vi "Power_spectrum.vi"(0 "U":dbl[](array[numeric]) format="%.2f", 2 "Sampling frequency":dbl format="%.2f", 3 "Spectrum input array":dbl[](array[numeric]) format="%.2f", 4 "Block No":i32=1) -> (5 "dF":dbl, 6 "SingleBlockSpectrum":dbl[](array[numeric]) format="%.2f", 7 "Spectrum Accumulator array":dbl[](array[numeric]) format="%.2f")   [LabVIEW 2015]
uses:
  <vilib>/Analysis/2dsp.llb/Power Spectrum (DBL).vi
  <vilib>/Analysis/baseanly.llb/Mean.vi
  <vilib>/Analysis/baseanly.llb/Mean (DBL).vi
  <vilib>/Analysis/NI_AALPro.lvlib
panel:
  out "size":i32
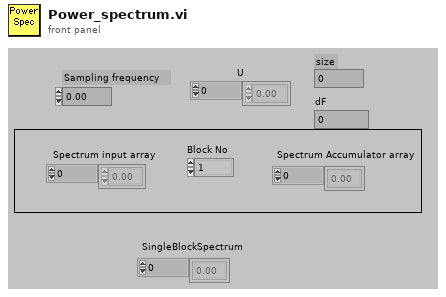
[diagram p1: front panel]
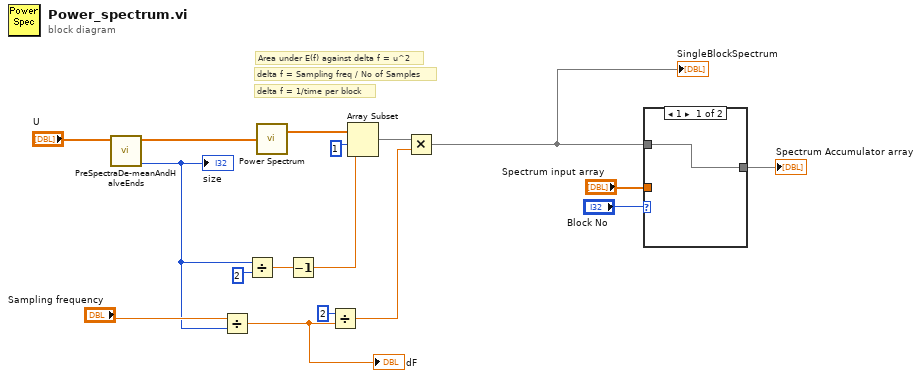
[diagram p0: block diagram]
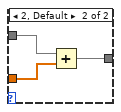
[diagram p2: hidden frame]
diagram:
  # "Area under E(f) against delta f = u^2"
  # "delta f = 1/time per block"
  # "delta f = Sampling freq / No of Samples"
  n1 = call "PreSpectraDe-meanAndHalveEnds.vi"("Array"="U") -> ("length"=w2:i32, "PreppedArray"=w14:dbl[])  [unwired: 9 in]
  "size" <- w2
  n2 = Divide(x="Sampling frequency", y=w2) -> (x/y=w9:dbl)
  "dF" <- w9
  n3 = Divide(x=w2, y=2) -> (x/y=w5:dbl)
  n4 = call-poly <vilib>:"Power Spectrum.vi"("X"=w14) -> ("Power Spectrum"=w15:dbl[])  [unwired: 1 out]
  n5 = Decrement(x=w5) -> (x-1=w4:dbl)
  n6 = Divide(x=2, y=w9) -> (x/y=w11:dbl)
  n7 = Array Subset(array=w15, index=1, length=w4) -> (w10:dbl[])
  n8 = Multiply(x=w10, y=w11) -> (x*y=w1:dbl[])
  "SingleBlockSpectrum" <- w1
  n9 = case shown="1" "Block No" {
    tunnel: [w18 w21] -> w3
    tunnel: w1 -> [w18 w20]
    tunnel: "Spectrum input array" -> [_ w19]
    frame 1 {
    }
    frame 2, Default {
      n10 = Add(x=w20, y=w19) -> (x+y=w21:dbl[])
    }
  }
  "Spectrum Accumulator array" <- w3
